vi "Case_String.vi"() -> ()   [LabVIEW 2016]
panel:
  in  "String":string
  out "Numeric Indicator":dbl
  in  "B":dbl
  in  "A":dbl
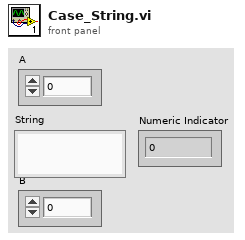
[diagram p1: front panel]
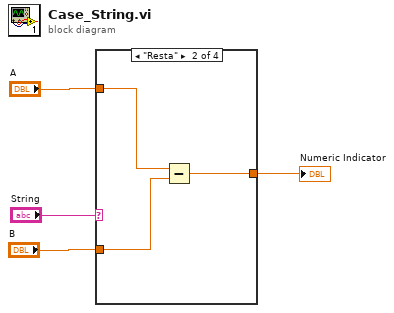
[diagram p0: block diagram]
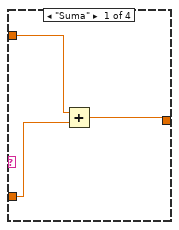
[diagram p2: hidden frame]
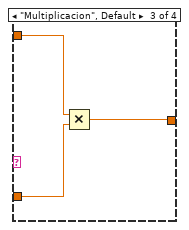
[diagram p3: hidden frame]
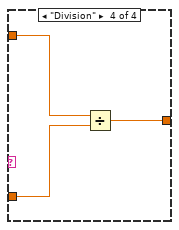
[diagram p4: hidden frame]
diagram:
  n1 = case shown="\"Resta\"" "String" {
    tunnel: "A" -> [w6 w10 w13 w14]
    tunnel: "B" -> [w5 w9 w12 w16]
    tunnel: [w7 w8 w11 w15] -> w2
    frame "Suma" {
      n2 = Add(x=w6, y=w5) -> (x+y=w7:dbl)
    }
    frame "Resta" {
      n3 = Subtract(x=w10, y=w9) -> (x-y=w8:dbl)
    }
    frame "Multiplicacion", Default {
      n4 = Multiply(x=w13, y=w12) -> (x*y=w11:dbl)
    }
    frame "Division" {
      n5 = Divide(x=w14, y=w16) -> (x/y=w15:dbl)
    }
  }
  "Numeric Indicator" <- w2
